vi "BuildCustomDashBoardData.vi"() -> ()   [LabVIEW 2013]
doc: "This VI builds data and sends it back to the dashboard PC program. By default it sends back the raw values for the first analog, digital, and solenoid module. Modify it to send back the data you want to view. Consider adding higher level data to the Dashboard Datatype.ctl and to this VI. Then update the Dashboard to display the data however you like.\n\nThis software is licensed. Open the labview\\readme\\WPI Robotics Library Open Source License.txt file for more information."
uses:
  typedefs/DashboardEnable.ctl
  typedefs/fg_typedef.ctl
  <vilib>/Rock Robotics/SystemInterfaces/Typedef/FPGA_TypedefDigitalModule.ctl
  typedefs/dash dio.ctl
  typedefs/misc dash data.ctl
  typedefs/dashboard safety status data.ctl
  typedefs/dash error type def.ctl
  <vilib>/Rock Robotics/SystemInterfaces/System/FPGA_SystemGet.vi
  <vilib>/NI_Real-Time Target Support.lvlib
  <vilib>/Rock Robotics/WPI/DriverStation/WPI_DriverStationDigitalData.ctl
  typedefs/subStates.ctl
  typedefs/custom dash data.ctl
  typedefs/Dashboard Datatype.ctl
panel:
  out "Errors":errorcluster
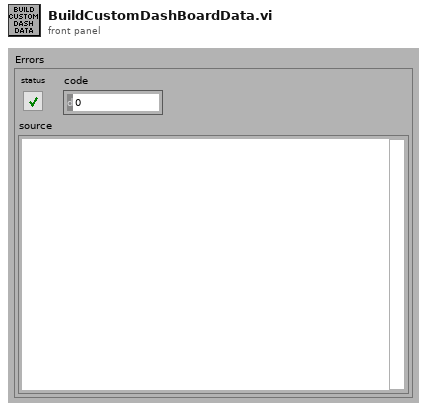
[diagram p1: front panel]
types:
  T1 = typedef "Dashboard Datatype.ctl" = cluster{cluster{"AnalogModule[0]":cluster{"Channel[0]":sgl, "Channel[1]":sgl, "Channel[2]":sgl, "Channel[3]":sgl, "Channel[4]":sgl, "Channel[5]":sgl, "Channel[6]":sgl, "Channel[7]":sgl}, "AnalogModule[1]":cluster{"Channel[0]":sgl, "Channel[1]":sgl, "Channel[2]":sgl, "Channel[3]":sgl, "Channel[4]":sgl, "Channel[5]":sgl, "Channel[6]":sgl, "Channel[7]":sgl}}, cluster{"DigitalModule[0]":T2, "DigitalModule[1]":T2}, "Solenoid":u8}
  T2 = typedef "WPI_DriverStationDigitalData.ctl" = cluster{"Relay Fwd":u8, "Relay Rev":u8, "GPIO":u16, "GPIO_OE":u16, "PWM":cluster{"PWM[0]":u8, "PWM[1]":u8, "PWM[2]":u8, "PWM[3]":u8, "PWM[4]":u8, "PWM[5]":u8, "PWM[6]":u8, "PWM[7]":u8, "PWM[8]":u8, "PWM[9]":u8}}
  T3 = typedef "custom dash data.ctl" = cluster{"Motors":cluster{"Pickup Motor":dbl, "Pickup Belt":dbl, "Pickup Distance ":dbl, "Pickup Rate":dbl, "Right Motor Rate":dbl, "Left Motor Rate":dbl, "Right Motor Distance":dbl, "Left Motor Distance":dbl}, "substates":cluster{"Latch":T4, "Pickup Arm":T4, "Belts":T4, "Shooter":T4, "Drive":T4}, "Safeties":cluster{"Arm Safety":bool, "Arm Limit":bool}, "Performance":cluster{"CPU Usage":dbl, "Vision mSPI":u32, "Main mSPI":u32}, "Vision Enabled?":bool, "Can Shoot Safely?":bool, "Timeout Error":cluster{"# of Timeouts":u32, "Time Out Error This Match":bool}, "Error FG Data":cluster{"Errors Present":bool, "Errors":string}, "Vision Data":cluster{"Hot Goal Present?":bool, "distance":dbl}}
  T4 = typedef "subStates.ctl" = enum16{"null", "wait", "driver control", "auto", "manual override", "hold position", "rotate", "pickup", "pass", "load", "goto shoot", "shoot high goal", "shoot low goal", "cancel arm", "cancel shooter", "end", "test"}
  T5 = typedef "fg_typedef.ctl" = enum16{"Get", "Set"}
  T6 = cluster{"# of Timeouts":u32, "Time Out Error This Match":bool}
  T7 = typedef "FPGA_TypedefDigitalModule.ctl" = enum16{"Digital Module 1", "Digital Module 2"}
  T8 = typedef "dash dio.ctl" = cluster{"Relay Forward":u8, "Relay Reverse":u8, u32, u32, cluster{"[0]":u8, "[1]":u8, "[2]":u8, "[3]":u8, "[4]":u8, "[5]":u8, "[6]":u8, "[7]":u8, "[8]":u8, "[9]":u8}}[]
  T9 = typedef "misc dash data.ctl" = cluster{"Total (%)":dbl, "Vision mSPI":u32, "Main mSPI":u32, "Vision":cluster{"Hot Goal Present?":bool, "distance":dbl}, "Enabled?":bool, "Safety Data":T10}
  T10 = typedef "dashboard safety status data.ctl" = cluster{"At Distance Limit":bool, "Encoder Error":bool, "Excedded Rate Limit":bool, "Encoder Directional Issue":bool}
  T11 = typedef "dash error type def.ctl" = cluster{"Error FG Data":cluster{"Errors Present":bool, "Errors":string}, "Timeout Data":cluster{"# of Timeouts":u32, "Time Out Error This Match":bool}, "Can Shoot Safely?":bool}
  T12 = typedef "DashboardEnable.ctl" = cluster{"Analog Module 1":bool[], "Analog Module 2":bool[], "Digital Module 1":bool, "Digital Module 2":bool, "Solenoid Module":bool}
  T13 = cluster{"AnalogModule[0]":cluster{"Channel[0]":sgl, "Channel[1]":sgl, "Channel[2]":sgl, "Channel[3]":sgl, "Channel[4]":sgl, "Channel[5]":sgl, "Channel[6]":sgl, "Channel[7]":sgl}, "AnalogModule[1]":cluster{"Channel[0]":sgl, "Channel[1]":sgl, "Channel[2]":sgl, "Channel[3]":sgl, "Channel[4]":sgl, "Channel[5]":sgl, "Channel[6]":sgl, "Channel[7]":sgl}}
  T14 = cluster{"DigitalModule[0]":T2, "DigitalModule[1]":T2}
  T15 = typedef "vision data.ctl" = cluster{"x":dbl, "y":dbl, "area":dbl, "width":dbl, "height":dbl, "Hot Goal Present?":bool, "distance":dbl}
  T16 = cluster{"Channel[0]":sgl, "Channel[1]":sgl, "Channel[2]":sgl, "Channel[3]":sgl, "Channel[4]":sgl, "Channel[5]":sgl, "Channel[6]":sgl, "Channel[7]":sgl}[]
  T17 = cluster{"Channel[0]":sgl, "Channel[1]":sgl, "Channel[2]":sgl, "Channel[3]":sgl, "Channel[4]":sgl, "Channel[5]":sgl, "Channel[6]":sgl, "Channel[7]":sgl}
  T18 = cluster{"AnalogModule[0][0]":sgl, "AnalogModule[0][1]":sgl, "AnalogModule[0][2]":sgl, "AnalogModule[0][3]":sgl, "AnalogModule[0][4]":sgl, "AnalogModule[0][5]":sgl, "AnalogModule[0][6]":sgl, "AnalogModule[0][7]":sgl}
  T19 = cluster{"[0]":cluster{"Channel[0]":sgl, "Channel[1]":sgl, "Channel[2]":sgl, "Channel[3]":sgl, "Channel[4]":sgl, "Channel[5]":sgl, "Channel[6]":sgl, "Channel[7]":sgl}, "[1]":cluster{"Channel[0]":sgl, "Channel[1]":sgl, "Channel[2]":sgl, "Channel[3]":sgl, "Channel[4]":sgl, "Channel[5]":sgl, "Channel[6]":sgl, "Channel[7]":sgl}}
  T20 = typedef "FPGA_DIODevRef.ctl" = cluster{"DevStatus":errorcluster, "Module":T7}
  T21 = cluster{"[0]":u8, "[1]":u8, "[2]":u8, "[3]":u8, "[4]":u8, "[5]":u8, "[6]":u8, "[7]":u8, "[8]":u8, "[9]":u8}
  T22 = typedef "FPGA_SolenoidDevRef.ctl" = cluster{"DevStatus":errorcluster, "Module":T23}
  T23 = typedef "FPGA_TypedefSolenoidModule.ctl" = enum16{"Solenoid Module 1", "Solenoid Module 2"}
  T24 = cluster{"Pickup Motor":dbl, "Pickup Belt":dbl, "Pickup Distance ":dbl, "Pickup Rate":dbl, "Right Motor Rate":dbl, "Left Motor Rate":dbl, "Right Motor Distance":dbl, "Left Motor Distance":dbl}
  T25 = cluster{"CPU Usage":dbl, "Vision mSPI":u32, "Main mSPI":u32}
  T26 = cluster{"Hot Goal Present?":bool, "distance":dbl}
  T27 = typedef "WPI_EncoderDevRef.ctl" = cluster{"DevStatus":errorcluster, "EncoderIndex":T28, "CounterIndex":T29, "DistancePerCount":dbl, "Decoding Type":T30}
  T28 = typedef "FPGA_EncoderIdx.ctl" = enum8{"Enc 0", "Enc 1", "Enc 2", "Enc 3", "Invalid"}
  T29 = typedef "FPGA_CounterCtrSystemIndex.ctl" = enum8{"Ctr 0", "Ctr 1", "Ctr 2", "Ctr 3", "Ctr 4", "Ctr 5", "Ctr 6", "Ctr 7", "Invalid"}
  T30 = typedef "WPI_EncoderType.ctl" = enum16{"1x", "2x", "4x"}
  T31 = typedef "WPI_MotorControlDeviceRef.ctl" = cluster{"DeviceStatus":errorcluster, "Type":enum16{"PWM", "CAN"}, "PWM":cluster{"Digital Module":T7, "PWM Channel":T32, "DeadBand":T33}, "CAN":cluster{"Device Number":u8, "Control Mode":T34, "Semaphore":T35, "Max Vout":dbl}, "Invert":bool, "TransformRef":T36, "InvTransformRef":T36}
  T32 = typedef "FPGA_DIOPWMChannel.ctl" = enum8{"PWM 1", "PWM 2", "PWM 3", "PWM 4", "PWM 5", "PWM 6", "PWM 7", "PWM 8", "PWM 9", "PWM 10", "Invalid"}
  T33 = typedef "WPI_PWMDeadband.ctl" = cluster{"Name":string, "maxPositivePwm":i32, "minPositivePwm":i32, "centerPwm":i32, "maxNegativePwm":i32, "minNegativePwm":i32, "angularRange":u16}
  T34 = typedef "WPI_CANJaguar_ControlMode.ctl" = enum8{"Percent VBus", "Current", "Speed", "Position", "Voltage"}
  T35 = typedef "Semaphore RefNum" = refnum<k1>
  T36 = typedef "WPI_PWMTransform_ConPane.ctl" = refnum<vi>
  T37 = typedef "NI_Real-Time Target Support.lvlib/RT CPU Load.ctl" = cluster{"Total (%)":dbl, "Time Critical (%)":dbl, "Timed Structures (%)":dbl, "High (%)":dbl, "Above Normal (%)":dbl, "Normal (%)":dbl, "Background (%)":dbl, "Idle (%)":dbl, "ISR (%)":dbl}
  T38 = cluster{"Vision mSPI":u32, "Main mSPI":u32, "Dash mSPI":u32}
  T39 = cluster{"Relay Forward":u8, "Relay Reverse":u8, u32, u32, cluster{"[0]":u8, "[1]":u8, "[2]":u8, "[3]":u8, "[4]":u8, "[5]":u8, "[6]":u8, "[7]":u8, "[8]":u8, "[9]":u8}}
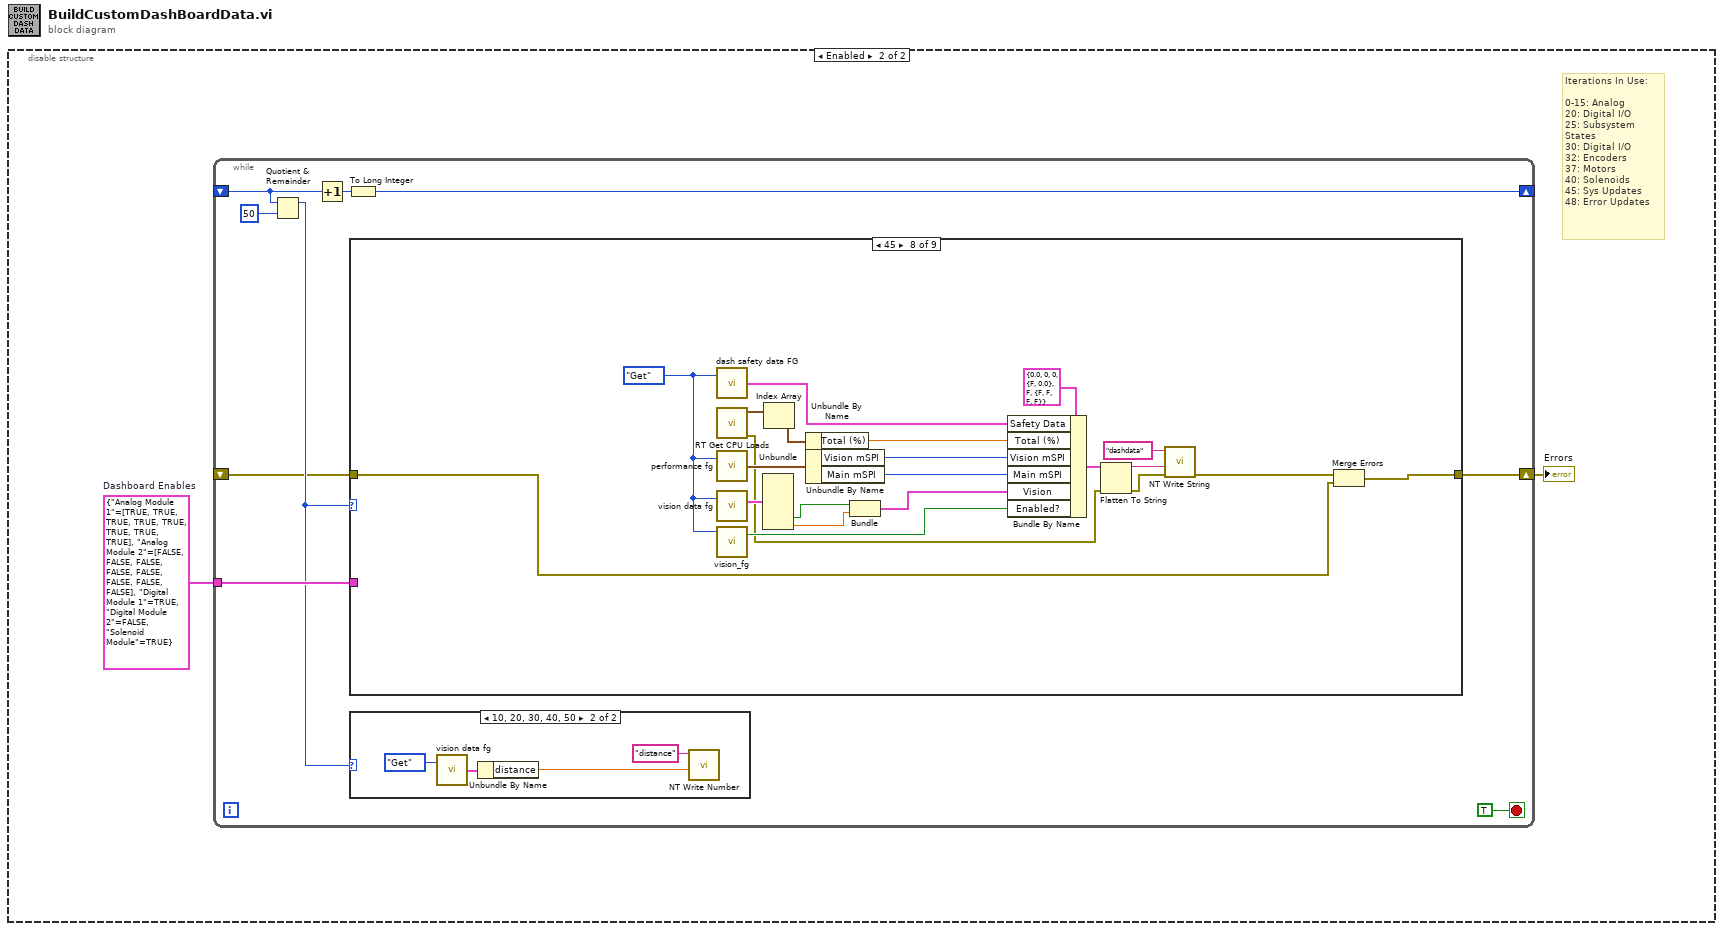
[diagram p0: block diagram]
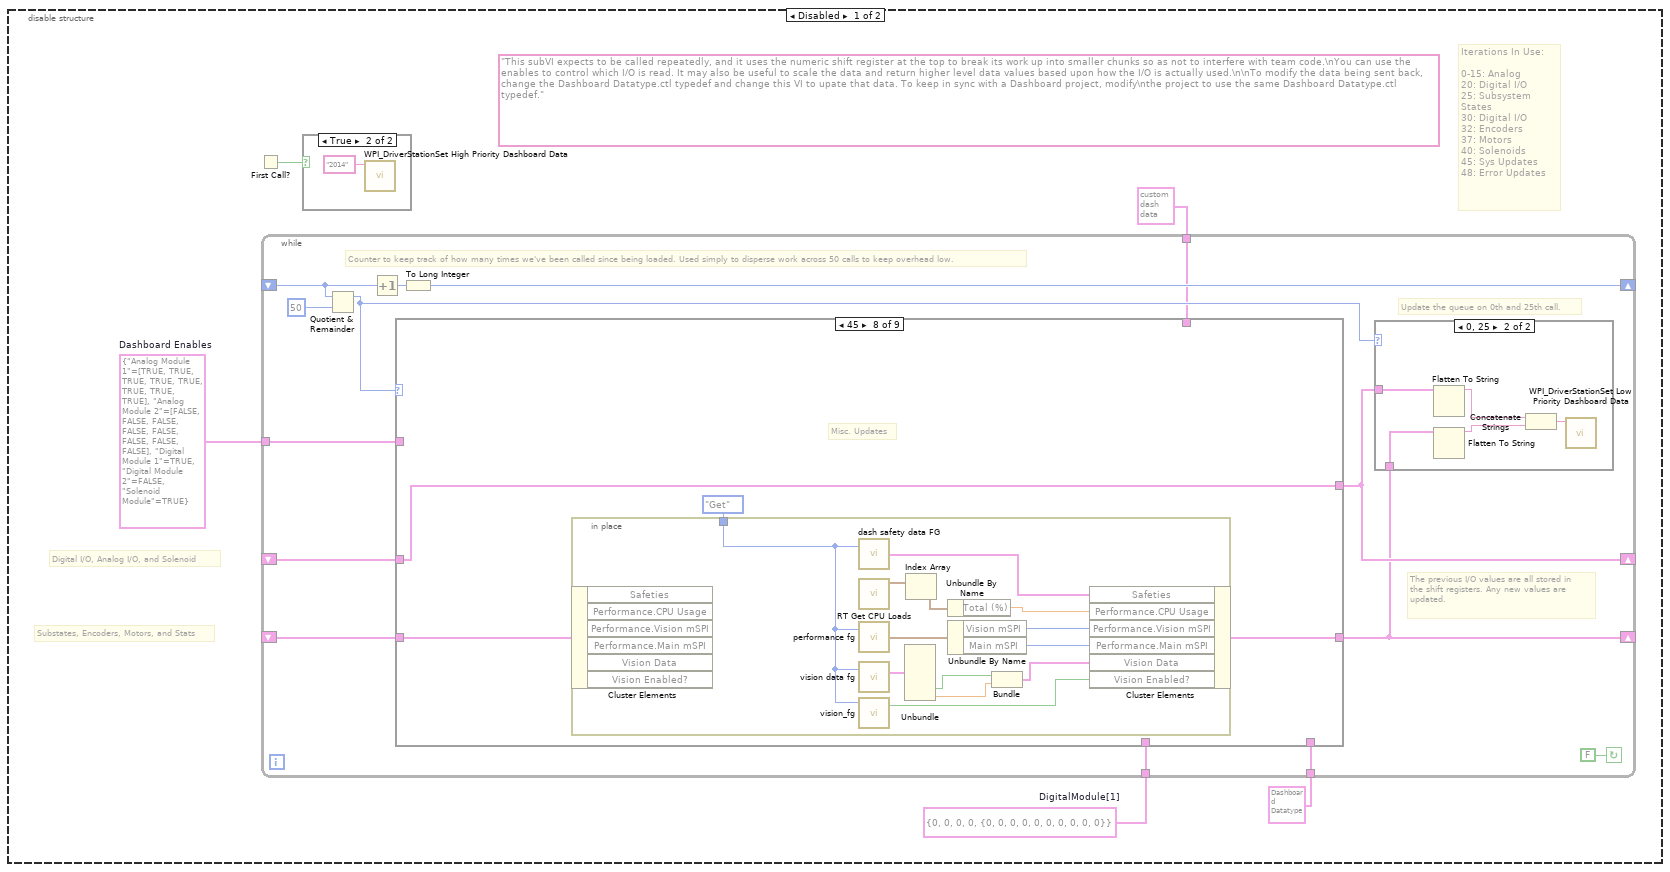
[diagram p2: hidden frame]
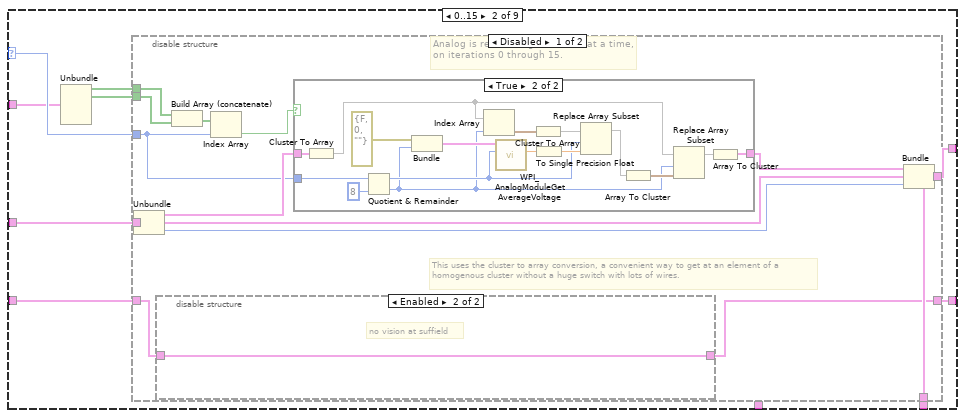
[diagram p6: hidden frame]
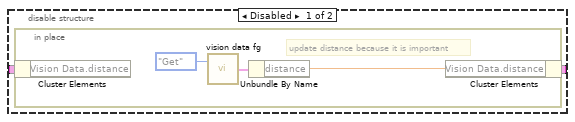
[diagram p8: hidden frame]
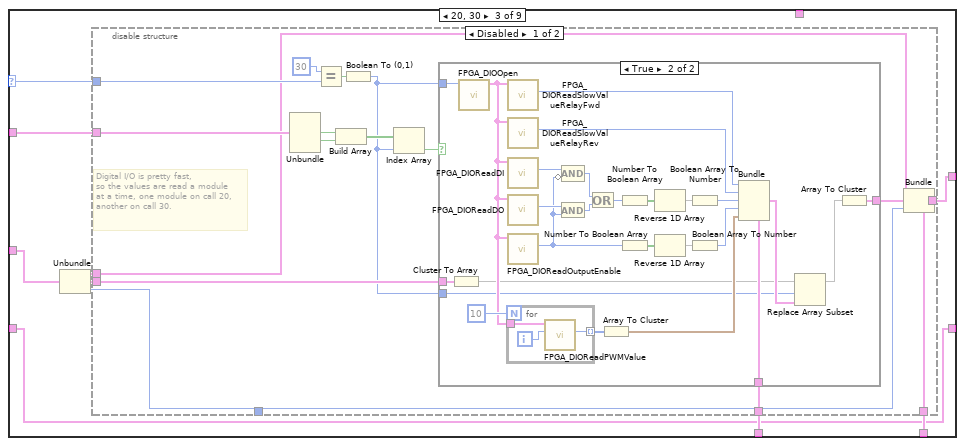
[diagram p10: hidden frame]
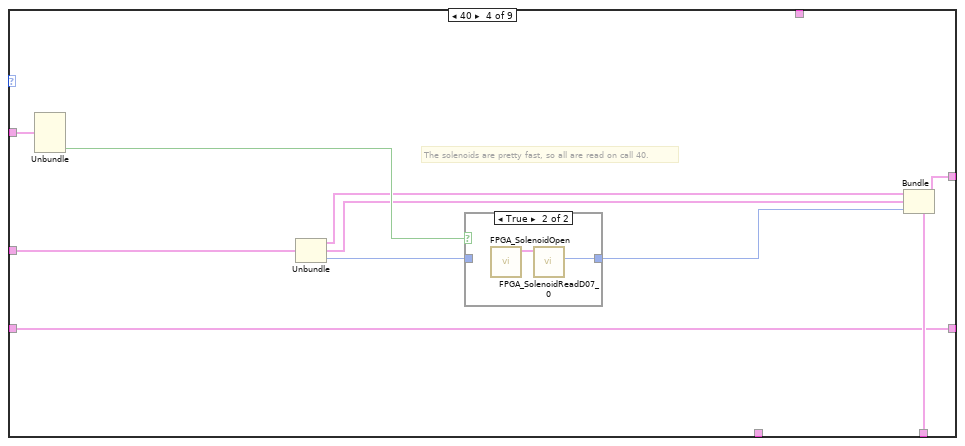
[diagram p13: hidden frame]
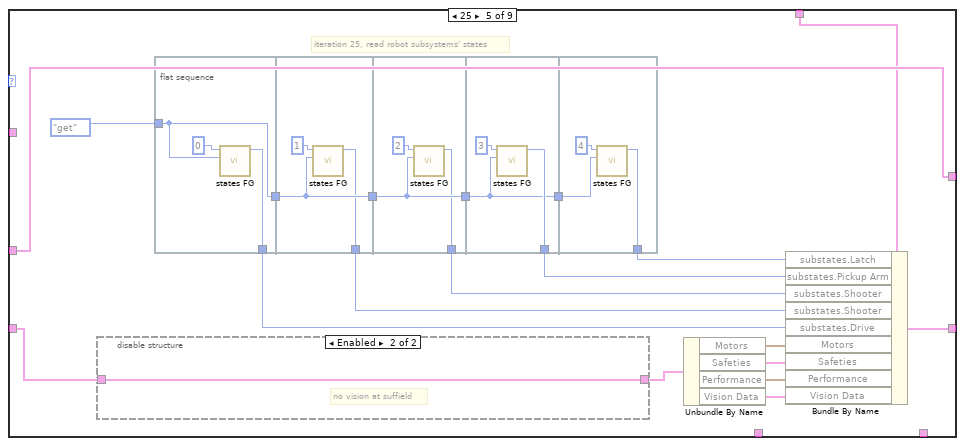
[diagram p15: hidden frame]
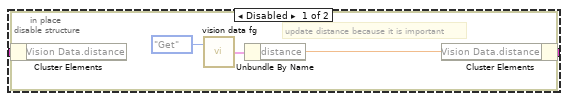
[diagram p16: hidden frame]
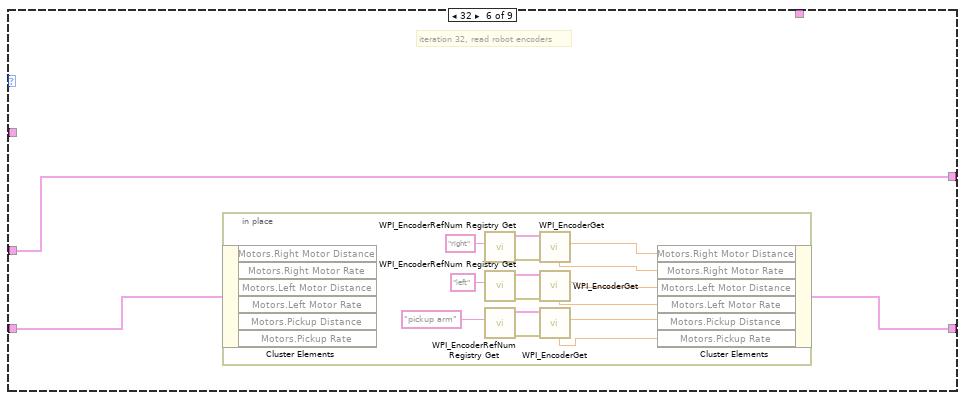
[diagram p17: hidden frame]
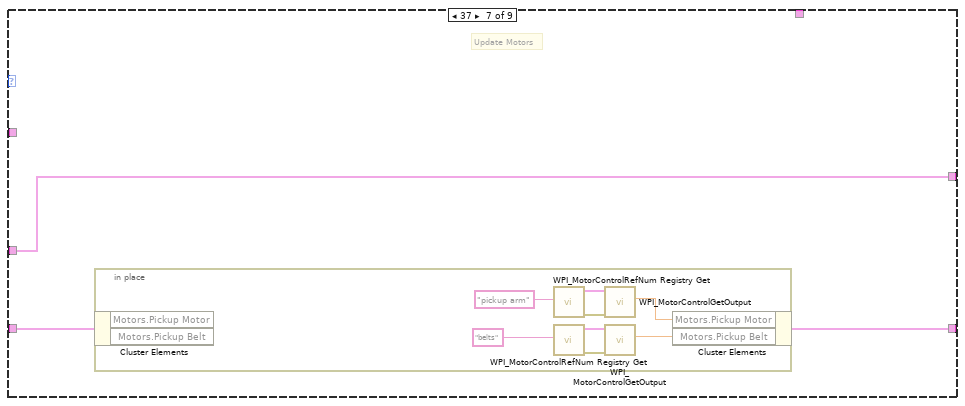
[diagram p18: hidden frame]
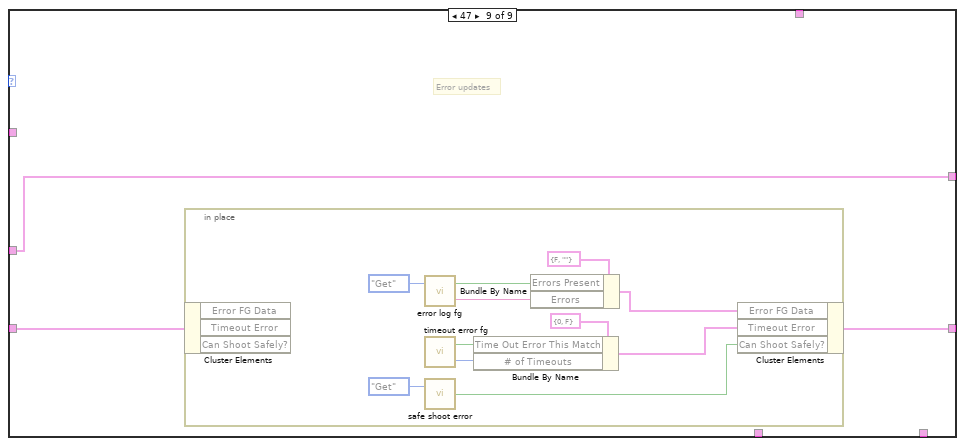
[diagram p19: hidden frame]
diagram:
  n1 = disable-structure shown="Enabled" {
    frame Disabled {
      w1 = T12 {"Analog Module 1"=[TRUE, TRUE, TRUE, TRUE, TRUE, TRUE, TRUE, TRUE], "Analog Module 2"=[FALSE, FALSE, FALSE, FALSE, FALSE, FALSE, FALSE, FALSE], "Digital Module 1"=TRUE, "Digital Module 2"=FALSE, "Solenoid Module"=TRUE}  # Dashboard Enables
      w2 = T2 {"Relay Fwd"=0, "Relay Rev"=0, "GPIO"=0, "GPIO_OE"=0, "PWM"={"PWM[0]"=0, "PWM[1]"=0, "PWM[2]"=0, "PWM[3]"=0, "PWM[4]"=0, "PWM[5]"=0, "PWM[6]"=0, "PWM[7]"=0, "PWM[8]"=0, "PWM[9]"=0}}  # DigitalModule[1]
      (unwired) "This subVI expects to be called repeatedly, and it uses the numeric shift register at the top to break its work up into smaller chunks so as not to interfere with team code.\nYou can use the enables to control which I/O is read. It may also be useful to scale the data and return higher level data values based upon how the I/O is actually used.\n\nTo modify the data being sent back, change the Dashboard Datatype.ctl typedef and change this VI to upate that data. To keep in sync with a Dashboard project, modify\nthe project to use the same Dashboard Datatype.ctl typedef."
      # "Iterations In Use:\n\n0-15: Analog\n20: Digital I/O \n25: Subsystem States\n30: Digital I/O\n32: Encoders\n37: Motors\n40: Solenoids\n45: Sys Updates\n48: Error Updates"
      # "Substates, Encoders, Motors, and Stats"
      # "Digital I/O, Analog I/O, and Solenoid"
      n2 = First Call?() -> (First Call?: T/F=w3:bool)
      n3 = while {
        shift-right: [w13] -> _
        shift-left: _ -> [w15]
        shift-right: [w10] -> _
        shift-left: _ -> [w18]
        tunnel: w2 -> [w17]
        tunnel: T1 {{"AnalogModule[0]"={"Channel[0]"=0.0, "Channel[1]"=0.0, "Channel[2]"=0.0, "Channel[3]"=0.0, "Channel[4]"=0.0, "Channel[5]"=0.0, "Channel[6]"=0.0, "Channel[7]"=0.0}, "AnalogModule[1]"={"Channel[0]"=0.0, "Channel[1]"=0.0, "Channel[2]"=0.0, "Channel[3]"=0.0, "Channel[4]"=0.0, "Channel[5]"=0.0, "Channel[6]"=0.0, "Channel[7]"=0.0}}, {"DigitalModule[0]"={"Relay Fwd"=0, "Relay Rev"=0, "GPIO"=0, "GPIO_OE"=0, "PWM"={"PWM[0]"=0, "PWM[1]"=0, "PWM[2]"=0, "PWM[3]"=0, "PWM[4]"=0, "PWM[5]"=0, "PWM[6]"=0, "PWM[7]"=0, "PWM[8]"=0, "PWM[9]"=0}}, "DigitalModule[1]"={"Relay Fwd"=0, "Relay Rev"=0, "GPIO"=0, "GPIO_OE"=0, "PWM"={"PWM[0]"=0, "PWM[1]"=0, "PWM[2]"=0, "PWM[3]"=0, "PWM[4]"=0, "PWM[5]"=0, "PWM[6]"=0, "PWM[7]"=0, "PWM[8]"=0, "PWM[9]"=0}}}, "Solenoid"=0} ("Dashboard Data") -> [w12]
        tunnel: w1 -> [w11]
        shift-right: [w7] -> _
        shift-left: _ -> [w8]
        tunnel: T3 {"Motors"={"Pickup Motor"=0.0, "Pickup Belt"=0.0, "Pickup Distance "=0.0, "Pickup Rate"=0.0, "Right Motor Rate"=0.0, "Left Motor Rate"=0.0, "Right Motor Distance"=0.0, "Left Motor Distance"=0.0}, "substates"={"Latch"=enum."null", "Pickup Arm"=enum."null", "Belts"=enum."null", "Shooter"=enum."null", "Drive"=enum."null"}, "Safeties"={"Arm Safety"=FALSE, "Arm Limit"=FALSE}, "Performance"={"CPU Usage"=0.0, "Vision mSPI"=0, "Main mSPI"=0}, "Vision Enabled?"=FALSE, "Can Shoot Safely?"=FALSE, "Timeout Error"={"# of Timeouts"=0, "Time Out Error This Match"=FALSE}, "Error FG Data"={"Errors Present"=FALSE, "Errors"=""}, "Vision Data"={"Hot Goal Present?"=FALSE, "distance"=0.0}} ("Custom Dash Data") -> [w9]
        stop <- FALSE continue-if-true
        # "Counter to keep track of how many times we've been called since being loaded. Used simply to disperse work across 50 calls to keep overhead low."
        # "Update the queue on 0th and 25th call."
        # "The previous I/O values are all stored in\nthe shift registers. Any new values are\nupdated."
        n4 = Quotient & Remainder(x=w15, y=50) -> (x-y*floor(x/y)=w14:i32)  [unwired: 1 out]
        n5 = Increment(x=w15) -> (x+1=w20:i32)
        n6 = case shown="45" w14 {
          selector: w14 -> [_ w35 w82 _ _ _ _ _ _]
          tunnel: [w27 w31 w77 w136 w151 w184 w203 w214 w230] -> w10
          tunnel: w18 -> [w27 w30 w79 w138 w151 w184 w203 w214 w230]
          tunnel: w17 -> [_ _ w83 _ _ _ _ _ _]
          tunnel: w12 -> [_ w36 w78 w135 _ _ _ _ _]
          tunnel: w11 -> [_ w34 w81 w139 _ _ _ _ _]
          tunnel: w9 -> [_ _ _ _ w149 _ _ _ _]
          tunnel: [w26 w28 w76 w132 w150 w185 w202 w215 w231] -> w7
          tunnel: w8 -> [w26 w29 w76 w132 w145 w183 w201 w213 w229]
          frame Default {
            # "Don't update any I/O"
          }
          frame 0..15 {
            n7 = Unbundle(w34) -> ("Analog Module 1"=w33:bool[], "Analog Module 2"=w32:bool[])  [unwired: 3 out]
            n8 = disable-structure shown="Disabled" {
              disable-tunnel: w36 -> [w47 _]
              disable-tunnel: w35 -> [w45 _]
              disable-tunnel: w33 -> [w44 _]
              disable-tunnel: w32 -> [w43 _]
              disable-tunnel: [w42 _] -> w31
              disable-tunnel: w30 -> [w41 _]
              disable-tunnel: w29 -> [w38 _]
              disable-tunnel: [w37 _] -> w28
              frame Disabled {
                # "This uses the cluster to array conversion, a convenient way to get at an element of a\nhomogenous cluster without a huge switch with lots of wires."
                # "Analog is read a single channel at a time,\non iterations 0 through 15."
                n9 = Unbundle(w41) -> (w46:T13, w40:T14, "Solenoid"=w39:u8)
                n10 = disable-structure shown="Enabled" {
                  disable-tunnel: w38 -> [w69 w73]
                  disable-tunnel: [w68 w73] -> w37
                  frame Disabled {
                    n11 = in-place {
                      # "update distance because it is important"
                      n12 = in-place-cluster #1(w69) -> ()  [unwired: 1 out]
                      n13 = call "vision data fg.vi"("Menu"=fg_typedef."Get") -> ("Output"=w71:T15)  [unwired: 1 in]
                      n14 = Unbundle By Name(w71) -> ("distance"=w70:dbl)
                      n15 = in-place-cluster #1("Vision Data.distance"=w70) -> (w68:T3)
                    }
                  }
                  frame Enabled {
                    # "no vision at suffield"
                  }
                }
                n16 = Build Array (concatenate)(w44, w43) -> (w49:bool[])
                n17 = Index Array(array=w49, index=w45) -> (element=w50:bool)
                n18 = case shown="True" w50 {
                  tunnel: w45 -> [_ w58]
                  tunnel: [w51 w55] -> w48
                  tunnel: w46 -> [w51 w54]
                  frame False {
                  }
                  frame True {
                    n19 = Cluster To Array(cluster=w54) -> (array=w53:T16)
                    n20 = Quotient & Remainder(x=w58, y=8) -> (x-y*floor(x/y)=w57:i32, floor(x/y)=w52:i32)
                    n21 = Bundle("DevStatus"=errorcluster {"status"=FALSE, "code"=0, "source"=""}, w52) -> (w66:cluster{"DevStatus":errorcluster, i32})  [unwired: 1 out]
                    n22 = Index Array(array=w53, index=w52) -> (element=w60:T17)
                    n23 = call <vilib>:"WPI_AnalogModuleGetAverageVoltage.vi"("Channel"=w57, "AnalogModuleDevStatus"=w66) -> ("Average Voltage"=w63:dbl)  [unwired: 1 in, 8 out]
                    n24 = Cluster To Array(cluster=w60) -> (array=w59:sgl[])
                    n25 = To Single Precision Float(number=w63) -> (single precision float=w62:sgl)
                    n26 = Replace Array Subset(array=w59, new element=w62, index=w57) -> (w61:sgl[])
                    n27 = Array To Cluster(array=w61) -> (cluster=w65:T18)
                    n28 = Replace Array Subset(array=w53, new element=w65, index=w52) -> (w56:T16)
                    n29 = Array To Cluster(array=w56) -> (cluster=w55:T19)
                  }
                }
                n30 = Bundle(cluster=w47, w48, w40, "Solenoid"=w39) -> (w42:T1)
              }
              frame Enabled {
              }
            }
          }
          frame 20, 30 {
            n31 = Unbundle(w79) -> (w75:T13, w80:T14, "Solenoid"=w74:u8)
            n32 = disable-structure shown="Disabled" {
              disable-tunnel: w83 -> [w99 _]
              disable-tunnel: w82 -> [w95 _]
              disable-tunnel: w81 -> [w93 _]
              disable-tunnel: w80 -> [w90 _]
              disable-tunnel: w78 -> [w88 _]
              disable-tunnel: [w87 _] -> w77
              disable-tunnel: w75 -> [w85 _]
              disable-tunnel: w74 -> [w84 _]
              frame Disabled {
                # "Digital I/O is pretty fast,\nso the values are read a module\nat a time, one module on call 20,\nanother on call 30."
                n33 = Unbundle(w93) -> ("Digital Module 1"=w92:bool, "Digital Module 2"=w91:bool)  [unwired: 3 out]
                n34 = Equal?(x=30, y=w95) -> (x = y?=w97:bool)
                n35 = Build Array(w92, w91) -> (w94:bool[])
                n36 = Boolean To (0,1)(Boolean=w97) -> (0, 1=w86:i16)
                n37 = Index Array(array=w94, index=w86) -> (element=w96:bool)
                n38 = case shown="True" w96 {
                  tunnel: w99 -> [_ w108]
                  tunnel: [w100 w101] -> w89
                  tunnel: w86 -> [_ w106]
                  tunnel: w86 -> [_ w105]
                  tunnel: w90 -> [w100 w104]
                  frame False {
                  }
                  frame True {
                    n39 = Cluster To Array(cluster=w104) -> (array=w103:T2[])
                    n40 = call <vilib>:"FPGA_DIOOpen.vi"("Module (Module 1)"=w106) -> ("DIODeviceRef"=w124:T20)  [unwired: 1 in, 9 out]
                    n41 = for {
                      N: 10 -> [_]
                      tunnel: w124 -> [w129]
                      tunnel: [w127] -> w125 mode=indexing
                      i -> [w128]
                      n42 = call <vilib>:"FPGA_DIOReadPWMValue.vi"("PWMChannel"=w128, "DIODeviceRef In"=w129) -> ("PWMValue"=w127:u8)  [unwired: 1 in, 8 out]
                    }
                    n43 = call <vilib>:"FPGA_DIOReadSlowValueRelayFwd.vi"("DIODeviceRef In"=w124) -> ("Relay Forward"=w117:u8)  [unwired: 1 in, 9 out]
                    n44 = call <vilib>:"FPGA_DIOReadSlowValueRelayRev.vi"("DIODeviceRef In"=w124) -> ("Relay Reverse"=w118:u8)  [unwired: 1 in, 9 out]
                    n45 = call <vilib>:"FPGA_DIOReadDI.vi"("DIODeviceRef In"=w124) -> ("DI"=w122:u16)  [unwired: 1 in, 9 out]
                    n46 = call <vilib>:"FPGA_DIOReadDO.vi"("DIODeviceRef In"=w124) -> ("DO"=w121:u16)  [unwired: 1 in, 9 out]
                    n47 = call <vilib>:"FPGA_DIOReadOutputEnable.vi"("DIODeviceRef In"=w124) -> ("OutputEnable"=w112:u16)  [unwired: 1 in, 9 out]
                    n48 = And(x=w121, y=w112) -> (x .and. y?=w120:u16)
                    n49 = Compound Arithmetic op=AND(w122, invert w112) -> (w119:u16)
                    n50 = Or(x=w119, y=w120) -> (x .or. y?=w110:u16)
                    n51 = Array To Cluster(array=w125) -> (cluster=w123:T21)
                    n52 = Number To Boolean Array(number=w110) -> (Boolean array=w115:bool[])
                    n53 = Number To Boolean Array(number=w112) -> (Boolean array=w114:bool[])
                    n54 = Reverse 1D Array(array=w115) -> (reversed array=w116:bool[])
                    n55 = Reverse 1D Array(array=w114) -> (reversed array=w113:bool[])
                    n56 = Boolean Array To Number(Boolean array=w116) -> (number=w109:u32)
                    n57 = Boolean Array To Number(Boolean array=w113) -> (number=w111:u32)
                    n58 = Bundle(cluster=w108, "Relay Fwd"=w117, "Relay Rev"=w118, "GPIO"=w109, "GPIO_OE"=w111, "PWM"=w123) -> (w107:T2)
                    n59 = Replace Array Subset(array=w103, new element=w107, index=w105) -> (w102:T2[])
                    n60 = Array To Cluster(array=w102) -> (cluster=w101:cluster{"[0]":T2, "[1]":T2})
                  }
                }
                n61 = Bundle(cluster=w88, w85, w89, "Solenoid"=w84) -> (w87:T1)
              }
              frame Enabled {
              }
            }
          }
          frame 40 {
            # "The solenoids are pretty fast, so all are read on call 40."
            n62 = Unbundle(w139) -> ("Solenoid Module"=w133:bool)  [unwired: 4 out]
            n63 = Unbundle(w138) -> (w131:T13, w130:T14, "Solenoid"=w137:u8)
            n64 = case shown="True" w133 {
              tunnel: [w140 w141] -> w134
              tunnel: w137 -> [w140 _]
              frame False {
              }
              frame True {
                n65 = call <vilib>:"FPGA_SolenoidOpen.vi"() -> ("SolenoidDevRef"=w142:T22)  [unwired: 2 in, 9 out]
                n66 = call <vilib>:"FPGA_SolenoidReadD07_0.vi"("SolenoidDevRef"=w142) -> ("DO7:0"=w141:u8)  [unwired: 1 in, 9 out]
              }
            }
            n67 = Bundle(cluster=w135, w131, w130, "Solenoid"=w134) -> (w136:T1)
          }
          frame 25 {
            # "iteration 25, read robot subsystems' states"
            n68 = disable-structure shown="Enabled" {
              disable-tunnel: w145 -> [w163 w167]
              disable-tunnel: [w162 w167] -> w144
              frame Disabled {
                n69 = in-place {
                  # "update distance because it is important"
                  n70 = in-place-cluster #2(w163) -> ()  [unwired: 1 out]
                  n71 = call "vision data fg.vi"("Menu"=fg_typedef."Get") -> ("Output"=w165:T15)  [unwired: 1 in]
                  n72 = Unbundle By Name(w165) -> ("distance"=w164:dbl)
                  n73 = in-place-cluster #2("Vision Data.distance"=w164) -> (w162:T3)
                }
              }
              frame Enabled {
                # "no vision at suffield"
              }
            }
            n74 = flat-sequence {
              tunnel: enum16{"set", "get"}."get" ("menu (get)") -> [w170]
              tunnel: [w170] -> w158
              tunnel: [w168] -> w152
              tunnel: [w173] -> w159
              tunnel: w158 -> [w173]
              tunnel: [w171] -> w153
              tunnel: [w176] -> w160
              tunnel: w159 -> [w176]
              tunnel: [w174] -> w154
              tunnel: w160 -> [w177]
              tunnel: [w178] -> w155
              tunnel: [w177] -> w157
              tunnel: w157 -> [w181]
              tunnel: [w180] -> w156
              frame #0 {
                n75 = call "states FG.vi"("menu (get)"=w170, "Loop ID"=0) -> ("subState out"=w168:T4)  [unwired: 6 in, 3 out]
              }
              frame #1 {
                n76 = call "states FG.vi"("menu (get)"=w173, "Loop ID"=1) -> ("subState out"=w171:T4)  [unwired: 6 in, 3 out]
              }
              frame #2 {
                n77 = call "states FG.vi"("menu (get)"=w176, "Loop ID"=2) -> ("subState out"=w174:T4)  [unwired: 6 in, 3 out]
              }
              frame #3 {
                n78 = call "states FG.vi"("menu (get)"=w177, "Loop ID"=3) -> ("subState out"=w178:T4)  [unwired: 6 in, 3 out]
              }
              frame #4 {
                n79 = call "states FG.vi"("menu (get)"=w181, "Loop ID"=4) -> ("subState out"=w180:T4)  [unwired: 6 in, 3 out]
              }
            }
            n80 = Unbundle By Name(w144) -> ("Motors"=w143:T24, "Safeties"=w148:cluster{"Arm Safety":bool, "Arm Limit":bool}, "Performance"=w147:T25, "Vision Data"=w146:T26)
            n81 = Bundle By Name(cluster=w149, "substates.Latch"=w156, "substates.Pickup Arm"=w155, "substates.Shooter"=w154, "substates.Shooter"=w153, "substates.Drive"=w152, "Motors"=w143, "Safeties"=w148, "Performance"=w147, "Vision Data"=w146) -> (w150:T3)
          }
          frame 32 {
            # "iteration 32, read robot encoders"
            n82 = in-place {
              n83 = in-place-cluster #3(w183) -> ()  [unwired: 6 out]
              n84 = call <vilib>:"WPI_EncoderRefNum Registry Get.vi"("refnum name"="right") -> ("error out"=w192:errorcluster, "EncoderDevRef"=w193:T27)  [unwired: 9 in]
              n85 = call <vilib>:"WPI_EncoderRefNum Registry Get.vi"("refnum name"="left") -> ("error out"=w195:errorcluster, "EncoderDevRef"=w194:T27)  [unwired: 9 in]
              n86 = call <vilib>:"WPI_EncoderRefNum Registry Get.vi"("refnum name"="pickup arm") -> ("error out"=w199:errorcluster, "EncoderDevRef"=w200:T27)  [unwired: 9 in]
              n87 = call <vilib>:"WPI_EncoderGet.vi"("error in (no error)"=w192, "EncoderDevRef"=w193) -> ("Distance"=w187:dbl, "Rate"=w186:dbl)  [unwired: 4 in, 4 out]
              n88 = call <vilib>:"WPI_EncoderGet.vi"("error in (no error)"=w195, "EncoderDevRef"=w194) -> ("Distance"=w188:dbl, "Rate"=w189:dbl)  [unwired: 4 in, 4 out]
              n89 = call <vilib>:"WPI_EncoderGet.vi"("error in (no error)"=w199, "EncoderDevRef"=w200) -> ("Distance"=w197:dbl, "Rate"=w196:dbl)  [unwired: 4 in, 4 out]
              n90 = in-place-cluster #3("Motors.Right Motor Distance"=w187, "Motors.Right Motor Rate"=w186, "Motors.Left Motor Distance"=w188, "Motors.Left Motor Rate"=w189, "Motors.Pickup Distance"=w197, "Motors.Pickup Rate"=w196) -> (w185:T3)
            }
          }
          frame 37 {
            # "Update Motors"
            n91 = in-place {
              n92 = in-place-cluster #4(w201) -> ()  [unwired: 2 out]
              n93 = call <vilib>:"WPI_MotorControlRefNum Registry Get.vi"("refnum name"="pickup arm") -> ("error out"=w204:errorcluster, "MotorControlDevRef"=w208:T31)  [unwired: 9 in]
              n94 = call <vilib>:"WPI_MotorControlRefNum Registry Get.vi"("refnum name"="belts") -> ("error out"=w205:errorcluster, "MotorControlDevRef"=w211:T31)  [unwired: 9 in]
              n95 = call <vilib>:"WPI_MotorControlGetOutput.vi"("error in (no error)"=w204, "MotorControlDevRef"=w208) -> ("Output"=w207:dbl)  [unwired: 7 in, 2 out]
              n96 = call <vilib>:"WPI_MotorControlGetOutput.vi"("error in (no error)"=w205, "MotorControlDevRef"=w211) -> ("Output"=w206:dbl)  [unwired: 7 in, 2 out]
              n97 = in-place-cluster #4("Motors.Pickup Motor"=w207, "Motors.Pickup Belt"=w206) -> (w202:T3)
            }
          }
          frame 45 {
            # "Misc. Updates"
            n98 = in-place {
              in-place-border: fg_typedef."Get" ("Menu (Get)") -> [w220]
              n99 = in-place-cluster #5(w213) -> ()  [unwired: 6 out]
              n100 = call "dash safety data FG.vi"("Menu"=w220) -> ("Safety Data Out"=w222:T10)  [unwired: 1 in]
              n101 = call <vilib>:"RT Get CPU Loads.vi"() -> ("CPU loads"=w227:T37[])  [unwired: 10 in, 1 out]
              n102 = call "performance fg.vi"("Menu"=w220) -> ("Output"=w223:T38)  [unwired: 1 in]
              n103 = call "vision data fg.vi"("Menu"=w220) -> ("Output"=w219:T15)  [unwired: 1 in]
              n104 = call "vision_fg.vi"("Menu"=w220) -> ("Enabled?"=w221:bool)  [unwired: 2 in, 1 out]
              n105 = Unbundle(w219) -> ("Hot Goal Present?"=w218:bool, "distance"=w217:dbl)  [unwired: 5 out]
              n106 = Index Array(array=w227) -> (element=w228:T37)  [unwired: 1 in]
              n107 = Unbundle By Name(w228) -> ("Total (%)"=w226:dbl)
              n108 = Unbundle By Name(w223) -> ("Vision mSPI"=w225:u32, "Main mSPI"=w224:u32)
              n109 = Bundle("Hot Goal Present?"=w218, "distance"=w217) -> (w216:T26)  [unwired: 1 in]
              n110 = in-place-cluster #5("Safeties"=w222, "Performance.CPU Usage"=w226, "Performance.Vision mSPI"=w225, "Performance.Main mSPI"=w224, "Vision Data"=w216, "Vision Enabled?"=w221) -> (w215:T3)
            }
          }
          frame 47 {
            # "Error updates"
            n111 = in-place {
              n112 = in-place-cluster #6(w229) -> ()  [unwired: 3 out]
              n113 = call "error log fg.vi"("Log Mode"=enum16{"Get", "Set", "Clear"}."Get") -> ("Errors"=w235:string, "Errors Present"=w234:bool)  [unwired: 1 in]
              n114 = call "timeout error fg.vi"() -> ("# of Timeouts"=w241:u32, "Time Out Error This Match"=w240:bool)  [unwired: 2 in]
              n115 = call "safe shoot error.vi"("Menu"=fg_typedef."Get") -> ("Can Shoot Safely?"=w237:bool)  [unwired: 1 in]
              n116 = Bundle By Name(cluster=T6 {"# of Timeouts"=0, "Time Out Error This Match"=FALSE}, "Time Out Error This Match"=w240, "# of Timeouts"=w241) -> (w239:T6)
              n117 = Bundle By Name(cluster=cluster{"Errors Present":bool, "Errors":string} {"Errors Present"=FALSE, "Errors"=""}, "Errors Present"=w234, "Errors"=w235) -> (w232:cluster{"Errors Present":bool, "Errors":string})
              n118 = in-place-cluster #6("Error FG Data"=w232, "Timeout Error"=w239, "Can Shoot Safely?"=w237) -> (w231:T3)
            }
          }
        }
        n119 = To Long Integer(number=w20) -> (32bit integer=w13:i32)
        n120 = case shown="0, 25" w14 {
          tunnel: w10 -> [_ w25]
          tunnel: w7 -> [_ w23]
          frame Default {
          }
          frame 0, 25 {
            n121 = Flatten To String(anything=w25) -> (data string=w24:string)  [unwired: 1 in, 4 out]
            n122 = Flatten To String(anything=w23) -> (data string=w21:string)  [unwired: 1 in, 4 out]
            n123 = Concatenate Strings(w24, w21) -> (w22:string)
            n124 = call <vilib>:"WPI_DriverStationSet Low Priority Dashboard Data.vi"("User Data"=w22) -> ()  [unwired: 1 in, 10 out]
          }
        }
      }
      n125 = case shown="True" w3 {
        frame False {
        }
        frame True {
          n126 = call <vilib>:"WPI_DriverStationSet High Priority Dashboard Data.vi"("User Data"="2014") -> ()  [unwired: 10 in, 1 out]
        }
      }
    }
    frame Enabled {
      w244 = T12 {"Analog Module 1"=[TRUE, TRUE, TRUE, TRUE, TRUE, TRUE, TRUE, TRUE], "Analog Module 2"=[FALSE, FALSE, FALSE, FALSE, FALSE, FALSE, FALSE, FALSE], "Digital Module 1"=TRUE, "Digital Module 2"=FALSE, "Solenoid Module"=TRUE}  # Dashboard Enables
      # "Iterations In Use:\n\n0-15: Analog\n20: Digital I/O \n25: Subsystem States\n30: Digital I/O\n32: Encoders\n37: Motors\n40: Solenoids\n45: Sys Updates\n48: Error Updates"
      n127 = while {
        shift-right: [w250] -> _
        shift-left: _ -> [w251]
        tunnel: w244 -> [w248]
        shift-right: [w246] -> w243
        shift-left: _ -> [w245]
        stop <- TRUE stop-if-true
        n128 = Quotient & Remainder(x=w251, y=50) -> (x-y*floor(x/y)=w247:i32)  [unwired: 1 out]
        n129 = Increment(x=w251) -> (x+1=w252:i32)
        n130 = To Long Integer(number=w252) -> (32bit integer=w250:i32)
        n131 = case shown="45" w247 {
          selector: w247 -> [_ w262 _ w315 _ _ _ _ _]
          tunnel: w248 -> [_ w265 _ w314 _ _ w397 _ _]
          tunnel: [w258 w260 w285 w305 w358 w380 w390 w408 w430] -> w246
          tunnel: w245 -> [w258 w259 w284 w306 w357 w379 w386 w407 w428]
          frame Default {
          }
          frame 0..15 {
            # "Analog is read a single channel at a time,\non iterations 0 through 15."
            n132 = Unbundle(w265) -> ("Analog Module 1"=w266:bool[], "Analog Module 2"=w267:bool[])  [unwired: 3 out]
            n133 = Build Array (concatenate)(w266, w267) -> (w263:bool[])
            n134 = Index Array(array=w263, index=w262) -> (element=w264:bool)
            n135 = case shown="True" w264 {
              tunnel: w262 -> [_ w279]
              tunnel: [w268 w269] -> w261
              tunnel: w259 -> [w268 _]
              frame False {
              }
              frame True {
                n136 = Quotient & Remainder(x=w279, y=8) -> (x-y*floor(x/y)=w276:i32, floor(x/y)=w280:i32)
                n137 = Bundle("DevStatus"=errorcluster {"status"=FALSE, "code"=0, "source"=""}, w280) -> (w282:cluster{"DevStatus":errorcluster, i32})  [unwired: 1 out]
                n138 = call <vilib>:"NT Read Numeric Array.vi"("Name"="analog") -> ("error out"=w271:errorcluster, "Numeric Array"=w277:dbl[])  [unwired: 9 in]
                n139 = call <vilib>:"WPI_AnalogModuleGetAverageVoltage.vi"("Channel"=w276, "AnalogModuleDevStatus"=w282) -> ("error out"=w270:errorcluster, "Average Voltage"=w275:dbl)  [unwired: 1 in, 7 out]
                n140 = Replace Array Subset(array=w277, new element=w275, index=w276) -> (w273:dbl[])
                n141 = Merge Errors(w271, w270) -> (w272:errorcluster)
                n142 = call <vilib>:"NT Write Numeric Array.vi"("error in"=w272, "Numeric Array"=w273, "Name"="analog") -> ("error out"=w269:errorcluster)  [unwired: 8 in]
              }
            }
            n143 = Merge Errors(w261, w259) -> (w260:errorcluster)
          }
          frame 25 {
            w299 = enum16{"set", "get"}."get" ("menu (get)")
            # "update subsystem states"
            n144 = call "states FG.vi"("menu (get)"=w299, "Loop ID"=0) -> ("subState out"=w296:T4)  [unwired: 6 in, 3 out]
            n145 = call "states FG.vi"("menu (get)"=w299, "Loop ID"=1) -> ("subState out"=w297:T4)  [unwired: 6 in, 3 out]
            n146 = call "states FG.vi"("menu (get)"=w299, "Loop ID"=2) -> ("subState out"=w298:T4)  [unwired: 6 in, 3 out]
            n147 = call "states FG.vi"("menu (get)"=w299, "Loop ID"=3) -> ("subState out"=w295:T4)  [unwired: 6 in, 3 out]
            n148 = call "states FG.vi"("menu (get)"=w299, "Loop ID"=4) -> ("subState out"=w294:T4)  [unwired: 6 in, 3 out]
            n149 = To Double Precision Float(number=w296) -> (double precision float=w292:dbl)
            n150 = To Double Precision Float(number=w297) -> (double precision float=w291:dbl)
            n151 = To Double Precision Float(number=w298) -> (double precision float=w290:dbl)
            n152 = To Double Precision Float(number=w295) -> (double precision float=w289:dbl)
            n153 = To Double Precision Float(number=w294) -> (double precision float=w288:dbl)
            n154 = Build Array(w292, w291, w290, w289, w288) -> (w287:dbl[])
            n155 = call <vilib>:"NT Write Numeric Array.vi"("Numeric Array"=w287, "Name"="subsystem_states") -> ("error out"=w286:errorcluster)  [unwired: 9 in]
            n156 = Merge Errors(w286, w284) -> (w285:errorcluster)
          }
          frame 20, 30 {
            # "Digital I/O is pretty fast,\nso the values are read a module\nat a time, one module on call 20,\nanother on call 30."
            n157 = Equal?(x=30, y=w315) -> (x = y?=w312:bool)
            n158 = Boolean To (0,1)(Boolean=w312) -> (0, 1=w313:i16)
            n159 = Unbundle(w314) -> ("Digital Module 1"=w317:bool, "Digital Module 2"=w316:bool)  [unwired: 3 out]
            n160 = To Long Integer(number=w313) -> (32bit integer=w310:i32)
            n161 = Select(t=FPGA_TypedefDigitalModule."Digital Module 1" ("Module (Module 1)"), s=w312, f=FPGA_TypedefDigitalModule."Digital Module 2" ("Module (Module 1)")) -> (s? t:f=w309:T7)
            n162 = Build Array(w317, w316) -> (w318:bool[])
            n163 = Index Array(array=w318, index=w310) -> (element=w319:bool)
            n164 = case shown="True" w319 {
              tunnel: w309 -> [_ w333]
              tunnel: w310 -> [_ w332]
              tunnel: [w321 w322] -> w307
              tunnel: w306 -> [w321 _]
              frame False {
              }
              frame True {
                n165 = call <vilib>:"FPGA_DIOOpen.vi"("Module (Module 1)"=w333) -> ("DIODeviceRef"=w350:T20)  [unwired: 1 in, 9 out]
                n166 = for {
                  N: 10 -> [_]
                  tunnel: w350 -> [w356]
                  tunnel: [w354] -> w351 mode=indexing
                  i -> [w355]
                  n167 = To Unsigned Byte Integer(number=w355) -> (unsigned 8bit integer=w353:u8)
                  n168 = call <vilib>:"FPGA_DIOReadPWMValue.vi"("PWMChannel"=w353, "DIODeviceRef In"=w356) -> ("PWMValue"=w354:u8)  [unwired: 1 in, 8 out]
                }
                n169 = call <vilib>:"FPGA_DIOReadSlowValueRelayFwd.vi"("DIODeviceRef In"=w350) -> ("Relay Forward"=w343:u8)  [unwired: 1 in, 9 out]
                n170 = call <vilib>:"FPGA_DIOReadSlowValueRelayRev.vi"("DIODeviceRef In"=w350) -> ("Relay Reverse"=w344:u8)  [unwired: 1 in, 9 out]
                n171 = call <vilib>:"FPGA_DIOReadDI.vi"("DIODeviceRef In"=w350) -> ("DI"=w348:u16)  [unwired: 1 in, 9 out]
                n172 = call <vilib>:"FPGA_DIOReadDO.vi"("DIODeviceRef In"=w350) -> ("DO"=w347:u16)  [unwired: 1 in, 9 out]
                n173 = call <vilib>:"FPGA_DIOReadOutputEnable.vi"("DIODeviceRef In"=w350) -> ("OutputEnable"=w338:u16)  [unwired: 1 in, 9 out]
                n174 = And(x=w347, y=w338) -> (x .and. y?=w346:u16)
                n175 = Compound Arithmetic op=AND(w348, invert w338) -> (w345:u16)
                n176 = Or(x=w345, y=w346) -> (x .or. y?=w336:u16)
                n177 = Number To Boolean Array(number=w336) -> (Boolean array=w341:bool[])
                n178 = Number To Boolean Array(number=w338) -> (Boolean array=w340:bool[])
                n179 = Reverse 1D Array(array=w341) -> (reversed array=w342:bool[])
                n180 = Reverse 1D Array(array=w340) -> (reversed array=w339:bool[])
                n181 = Array To Cluster(array=w351) -> (cluster=w349:T21)
                n182 = Boolean Array To Number(Boolean array=w342) -> (number=w335:u32)
                n183 = Boolean Array To Number(Boolean array=w339) -> (number=w337:u32)
                n184 = Bundle("Relay Forward"=w343, "Relay Reverse"=w344, w335, w337, w349) -> (w334:T39)  [unwired: 1 out]
                n185 = call <vilib>:"NT Read String.vi"("Name"="dio") -> ("error out"=w326:errorcluster, "String"=w325:string)  [unwired: 9 in]
                n186 = Unflatten From String(type=T8 [] ("array"), binary string=w325, error in (no error)=w326) -> (value=w323:T8)  [unwired: 2 in, 2 out]
                n187 = Replace Array Subset(array=w323, new element=w334, index=w332) -> (w331:T8)
                n188 = Flatten To String(anything=w331) -> (data string=w329:string, error out=w330:errorcluster)  [unwired: 1 in, 3 out]
                n189 = call <vilib>:"NT Write String.vi"("error in"=w330, "String"=w329, "Name"="dio") -> ("error out"=w322:errorcluster)  [unwired: 8 in]
              }
            }
            n190 = Merge Errors(w307, w306) -> (w305:errorcluster)
          }
          frame 32 {
            # "update encoders"
            n191 = call <vilib>:"WPI_EncoderRefNum Registry Get.vi"("refnum name"="pickup arm") -> ("error out"=w369:errorcluster, "EncoderDevRef"=w368:T27)  [unwired: 9 in]
            n192 = call <vilib>:"WPI_EncoderRefNum Registry Get.vi"("refnum name"="right") -> ("error out"=w374:errorcluster, "EncoderDevRef"=w373:T27)  [unwired: 9 in]
            n193 = call <vilib>:"WPI_EncoderRefNum Registry Get.vi"("refnum name"="left") -> ("error out"=w371:errorcluster, "EncoderDevRef"=w372:T27)  [unwired: 9 in]
            n194 = call <vilib>:"WPI_EncoderGet.vi"("error in (no error)"=w374, "EncoderDevRef"=w373) -> ("Distance"=w366:dbl, "Rate"=w365:dbl)  [unwired: 4 in, 4 out]
            n195 = call <vilib>:"WPI_EncoderGet.vi"("error in (no error)"=w371, "EncoderDevRef"=w372) -> ("Distance"=w364:dbl, "Rate"=w363:dbl)  [unwired: 4 in, 4 out]
            n196 = call <vilib>:"WPI_EncoderGet.vi"("error in (no error)"=w369, "EncoderDevRef"=w368) -> ("Distance"=w362:dbl, "Rate"=w361:dbl)  [unwired: 4 in, 4 out]
            n197 = Build Array(w366, w365, w364, w363, w362, w361) -> (w360:dbl[])
            n198 = call <vilib>:"NT Write Numeric Array.vi"("Numeric Array"=w360, "Name"="encoders") -> ("error out"=w359:errorcluster)  [unwired: 9 in]
            n199 = Merge Errors(w359, w357) -> (w358:errorcluster)
          }
          frame 37 {
            # "update motor array"
            n200 = call <vilib>:"WPI_MotorControlRefNum Registry Get.vi"("refnum name"="belts") -> ("error out"=w383:errorcluster, "MotorControlDevRef"=w385:T31)  [unwired: 9 in]
            n201 = call <vilib>:"WPI_MotorControlGetOutput.vi"("error in (no error)"=w383, "MotorControlDevRef"=w385) -> ("error out"=w378:errorcluster, "Output"=w382:dbl)  [unwired: 7 in, 1 out]
            n202 = call <vilib>:"NT Write Number.vi"("error in"=w378, "Numeric"=w382, "Name"="belts") -> ("error out"=w377:errorcluster)  [unwired: 8 in]
            n203 = Merge Errors(w379, w377) -> (w380:errorcluster)
          }
          frame 40 {
            # "The solenoids are pretty fast, so all are read on call 40."
            n204 = Unbundle(w397) -> ("Solenoid Module"=w398:bool)  [unwired: 4 out]
            n205 = call <vilib>:"NT Read Number.vi"("Name"="solenoids") -> ("error out"=w387:errorcluster, "Numeric"=w394:dbl)  [unwired: 9 in]
            n206 = To Unsigned Byte Integer(number=w394) -> (unsigned 8bit integer=w392:u8)
            n207 = case shown="True" w398 {
              tunnel: [w400 w404] -> w396
              tunnel: w392 -> [w400 _]
              tunnel: [w399 w402] -> w388
              tunnel: w387 -> [w399 w401]
              frame False {
              }
              frame True {
                n208 = call <vilib>:"FPGA_SolenoidOpen.vi"("error in (no error)"=w401) -> ("error out"=w403:errorcluster, "SolenoidDevRef"=w405:T22)  [unwired: 1 in, 8 out]
                n209 = call <vilib>:"FPGA_SolenoidReadD07_0.vi"("error in (no error)"=w403, "SolenoidDevRef"=w405) -> ("error out"=w402:errorcluster, "DO7:0"=w404:u8)  [unwired: 8 out]
              }
            }
            n210 = To Double Precision Float(number=w396) -> (double precision float=w391:dbl)
            n211 = call <vilib>:"NT Write Number.vi"("error in"=w388, "Numeric"=w391, "Name"="solenoids") -> ("error out"=w389:errorcluster)  [unwired: 8 in]
            n212 = Merge Errors(w389, w386) -> (w390:errorcluster)
          }
          frame 45 {
            w421 = fg_typedef."Get" ("Menu")
            n213 = call "dash safety data FG.vi"("Menu"=w421) -> ("Safety Data Out"=w406:T10)  [unwired: 1 in]
            n214 = call <vilib>:"RT Get CPU Loads.vi"() -> ("error out"=w410:errorcluster, "CPU loads"=w426:T37[])  [unwired: 10 in]
            n215 = call "performance fg.vi"("Menu"=w421) -> ("Output"=w425:T38)  [unwired: 1 in]
            n216 = call "vision data fg.vi"("Menu"=w421) -> ("Output"=w424:T15)  [unwired: 1 in]
            n217 = call "vision_fg.vi"("Menu"=w421) -> ("Enabled?"=w419:bool)  [unwired: 2 in, 1 out]
            n218 = Unbundle(w424) -> ("Hot Goal Present?"=w423:bool, "distance"=w422:dbl)  [unwired: 5 out]
            n219 = Index Array(array=w426) -> (element=w427:T37)  [unwired: 1 in]
            n220 = Unbundle By Name(w427) -> ("Total (%)"=w415:dbl)
            n221 = Unbundle By Name(w425) -> ("Vision mSPI"=w416:u32, "Main mSPI"=w417:u32)
            n222 = Bundle("Hot Goal Present?"=w423, "distance"=w422) -> (w418:T26)  [unwired: 1 in]
            n223 = Bundle By Name(cluster=T9 {"Total (%)"=0.0, "Vision mSPI"=0, "Main mSPI"=0, "Vision"={"Hot Goal Present?"=FALSE, "distance"=0.0}, "Enabled?"=FALSE, "Safety Data"={"At Distance Limit"=FALSE, "Encoder Error"=FALSE, "Excedded Rate Limit"=FALSE, "Encoder Directional Issue"=FALSE}}, "Safety Data"=w406, "Total (%)"=w415, "Vision mSPI"=w416, "Main mSPI"=w417, "Vision"=w418, "Enabled?"=w419) -> (w412:T9)
            n224 = Flatten To String(anything=w412, error in (no error)=w410) -> (data string=w414:string, error out=w411:errorcluster)  [unwired: 3 out]
            n225 = call <vilib>:"NT Write String.vi"("error in"=w411, "String"=w414, "Name"="dashdata") -> ("error out"=w409:errorcluster)  [unwired: 8 in]
            n226 = Merge Errors(w409, w407) -> (w408:errorcluster)
          }
          frame 47 {
            n227 = call "error log fg.vi"("Log Mode"=enum16{"Get", "Set", "Clear"}."Get") -> ("Errors"=w441:string, "Errors Present"=w440:bool)  [unwired: 1 in]
            n228 = call "timeout error fg.vi"() -> ("# of Timeouts"=w445:u32, "Time Out Error This Match"=w444:bool)  [unwired: 2 in]
            n229 = call "safe shoot error.vi"("Menu"=fg_typedef."Get") -> ("Can Shoot Safely?"=w436:bool)  [unwired: 1 in]
            n230 = Bundle By Name(cluster=T6 {"# of Timeouts"=0, "Time Out Error This Match"=FALSE}, "Time Out Error This Match"=w444, "# of Timeouts"=w445) -> (w437:T6)
            n231 = Bundle By Name(cluster=cluster{"Errors Present":bool, "Errors":string} {"Errors Present"=FALSE, "Errors"=""}, "Errors Present"=w440, "Errors"=w441) -> (w438:cluster{"Errors Present":bool, "Errors":string})
            n232 = Bundle By Name(cluster=T11 {"Error FG Data"={"Errors Present"=FALSE, "Errors"=""}, "Timeout Data"={"# of Timeouts"=0, "Time Out Error This Match"=FALSE}, "Can Shoot Safely?"=FALSE}, "Error FG Data"=w438, "Timeout Data"=w437, "Can Shoot Safely?"=w436) -> (w435:T11)
            n233 = Flatten To String(anything=w435) -> (data string=w431:string, error out=w433:errorcluster)  [unwired: 1 in, 3 out]
            n234 = call <vilib>:"NT Write String.vi"("error in"=w433, "String"=w431, "Name"="errors") -> ("error out"=w429:errorcluster)  [unwired: 8 in]
            n235 = Merge Errors(w429, w428) -> (w430:errorcluster)
          }
        }
        n236 = case shown="10, 20, 30, 40, 50" w247 {
          frame 0, Default {
          }
          frame 10, 20, 30, 40, 50 {
            n237 = call "vision data fg.vi"("Menu"=fg_typedef."Get") -> ("Output"=w256:T15)  [unwired: 1 in]
            n238 = Unbundle By Name(w256) -> ("distance"=w255:dbl)
            n239 = call <vilib>:"NT Write Number.vi"("Numeric"=w255, "Name"="distance") -> ()  [unwired: 9 in, 1 out]
          }
        }
      }
      "Errors" <- w243
    }
  }
